vi "Configure Load to Sequence - Single.vi"(8 "error in":errorcluster, 10 "measurement configuration":T6 {"Measurement timeout" format="%.3p"; "Load device voltage/current rating" format="%#_6pA"; "Load voltage/current setpoints" format="%#_6p"; "Load output function" items=["DC Voltage"=1006, "DC Current"=1007, "Pulse Voltage"=1049, "Pulse Current"=1050]; "Load sense" items=["Local"=1008, "Remote"=1009]; "Load transient response" items=["Slow"=1041, "Normal"=1038, "Fast"=1039, "Custom"=1042]; "Load current/voltage limit high" format="%#_6p"; "Load current/voltage limit low" format="%#_6p"; "Load current/voltage limit range" format="%#_6p"; "Load voltage/current level range" format="%#_6p"; "Power ON/Source voltage/current setpoints" format="%#_6p"; "Power ON/Source output function" items=["DC Voltage"=1006, "DC Current"=1007, "Pulse Voltage"=1049, "Pulse Current"=1050]; "Power ON/Source sense" items=["Local"=1008, "Remote"=1009]; "Source transient response" items=["Slow"=1041, "Normal"=1038, "Fast"=1039, "Custom"=1042]; "Source current/voltage limit high" format="%#_6p"; "Source current/voltage limit low" format="%#_6p"; "Power ON/Source current/voltage limit range" format="%#_6p"; "Source voltage/current level range" format="%#_6p"}, 11 "Waveform Mode - Control":T1={"Source Ganged Session Out"={"Ganged Config"=enum."Series", "Session List"=[], "Session Mode"=[], "Channel"=[]}, "Load Ganged Session Out"={"Ganged Config"=enum."Series", "Session List"=[], "Session Mode"=[], "Channel"=[]}, "Source Measure Record Length"=0, "Load Measure Record Length"=0, "Source Sequence Name"="", "Load Sequence Name"="", "Source First Sequence Call"=FALSE, "Load First Sequence Call"=FALSE, "Measurement Results"={"Source dt"=[], "Source voltages"=[], "Source currents"=[], "Ganged source voltages"=[], "Ganged source currents"=[0.0], "Load dt"=[], "Load voltages"=[], "Load currents"=[], "Ganged load voltages"=[], "Ganged load currents"=[], "Status"="", "Eload status"=""}, "No. of eload used"=0, "Measurement timeout"=0.0, "Load Source ON/OFF"=enum."SOURCE AND LOAD ON", "Load session out"="", "Source session out"="", "Load channel name"="", "Source channel name"="", "Source ganged/single"=FALSE, "Load ganged/single"=FALSE, "Source Master/Single resource name"="", "Source Slave resource name"=[], "Load Master/Single resource name"="", "Load Slave resource name"=[]}) -> (0 "error out":errorcluster, 3 "Waveform Mode - Results":T1={"Source Ganged Session Out"={"Ganged Config"=enum."Series", "Session List"=[], "Session Mode"=[], "Channel"=[]}, "Load Ganged Session Out"={"Ganged Config"=enum."Series", "Session List"=[], "Session Mode"=[], "Channel"=[]}, "Source Measure Record Length"=0, "Load Measure Record Length"=0, "Source Sequence Name"="", "Load Sequence Name"="", "Source First Sequence Call"=FALSE, "Load First Sequence Call"=FALSE, "Measurement Results"={"Source dt"=[], "Source voltages"=[], "Source currents"=[], "Ganged source voltages"=[], "Ganged source currents"=[0.0], "Load dt"=[], "Load voltages"=[], "Load currents"=[], "Ganged load voltages"=[], "Ganged load currents"=[], "Status"="", "Eload status"=""}, "No. of eload used"=0, "Measurement timeout"=0.0, "Load Source ON/OFF"=enum."SOURCE AND LOAD ON", "Load session out"="", "Source session out"="", "Load channel name"="", "Source channel name"="", "Source ganged/single"=FALSE, "Load ganged/single"=FALSE, "Source Master/Single resource name"="", "Source Slave resource name"=[], "Load Master/Single resource name"="", "Load Slave resource name"=[]})   [LabVIEW 2021, in "Waveform Mode_Channel Ganging.lvlib"]
doc: "Configure load to sequence"
uses:
  Measurement Configuration.ctl
  Controls/Waveform Mode Measurement.ctl
  shared subVIs/ctl/NIDCPower_channel_ganging - ctl - ganged session.ctl
  shared subVIs/ctl/NIDCPower_channel_ganging - ctl - ganged config.ctl
  shared subVIs/ctl/NIDCPower_channel_ganging - ctl - channel mode.ctl
  Measurement Results.ctl
  <instrlib>/niDCPower/nidcpower.llb/niDCPower Source Mode.ctl
  <instrlib>/niDCPower/nidcpower.llb/niDCPower Sequence Attribute Type.ctl
  <instrlib>/niDCPower/nidcpower.llb/niDCPower Create Advanced Sequence Step With Channels.vi
  Waveform Mode_Channel Ganging.lvlib
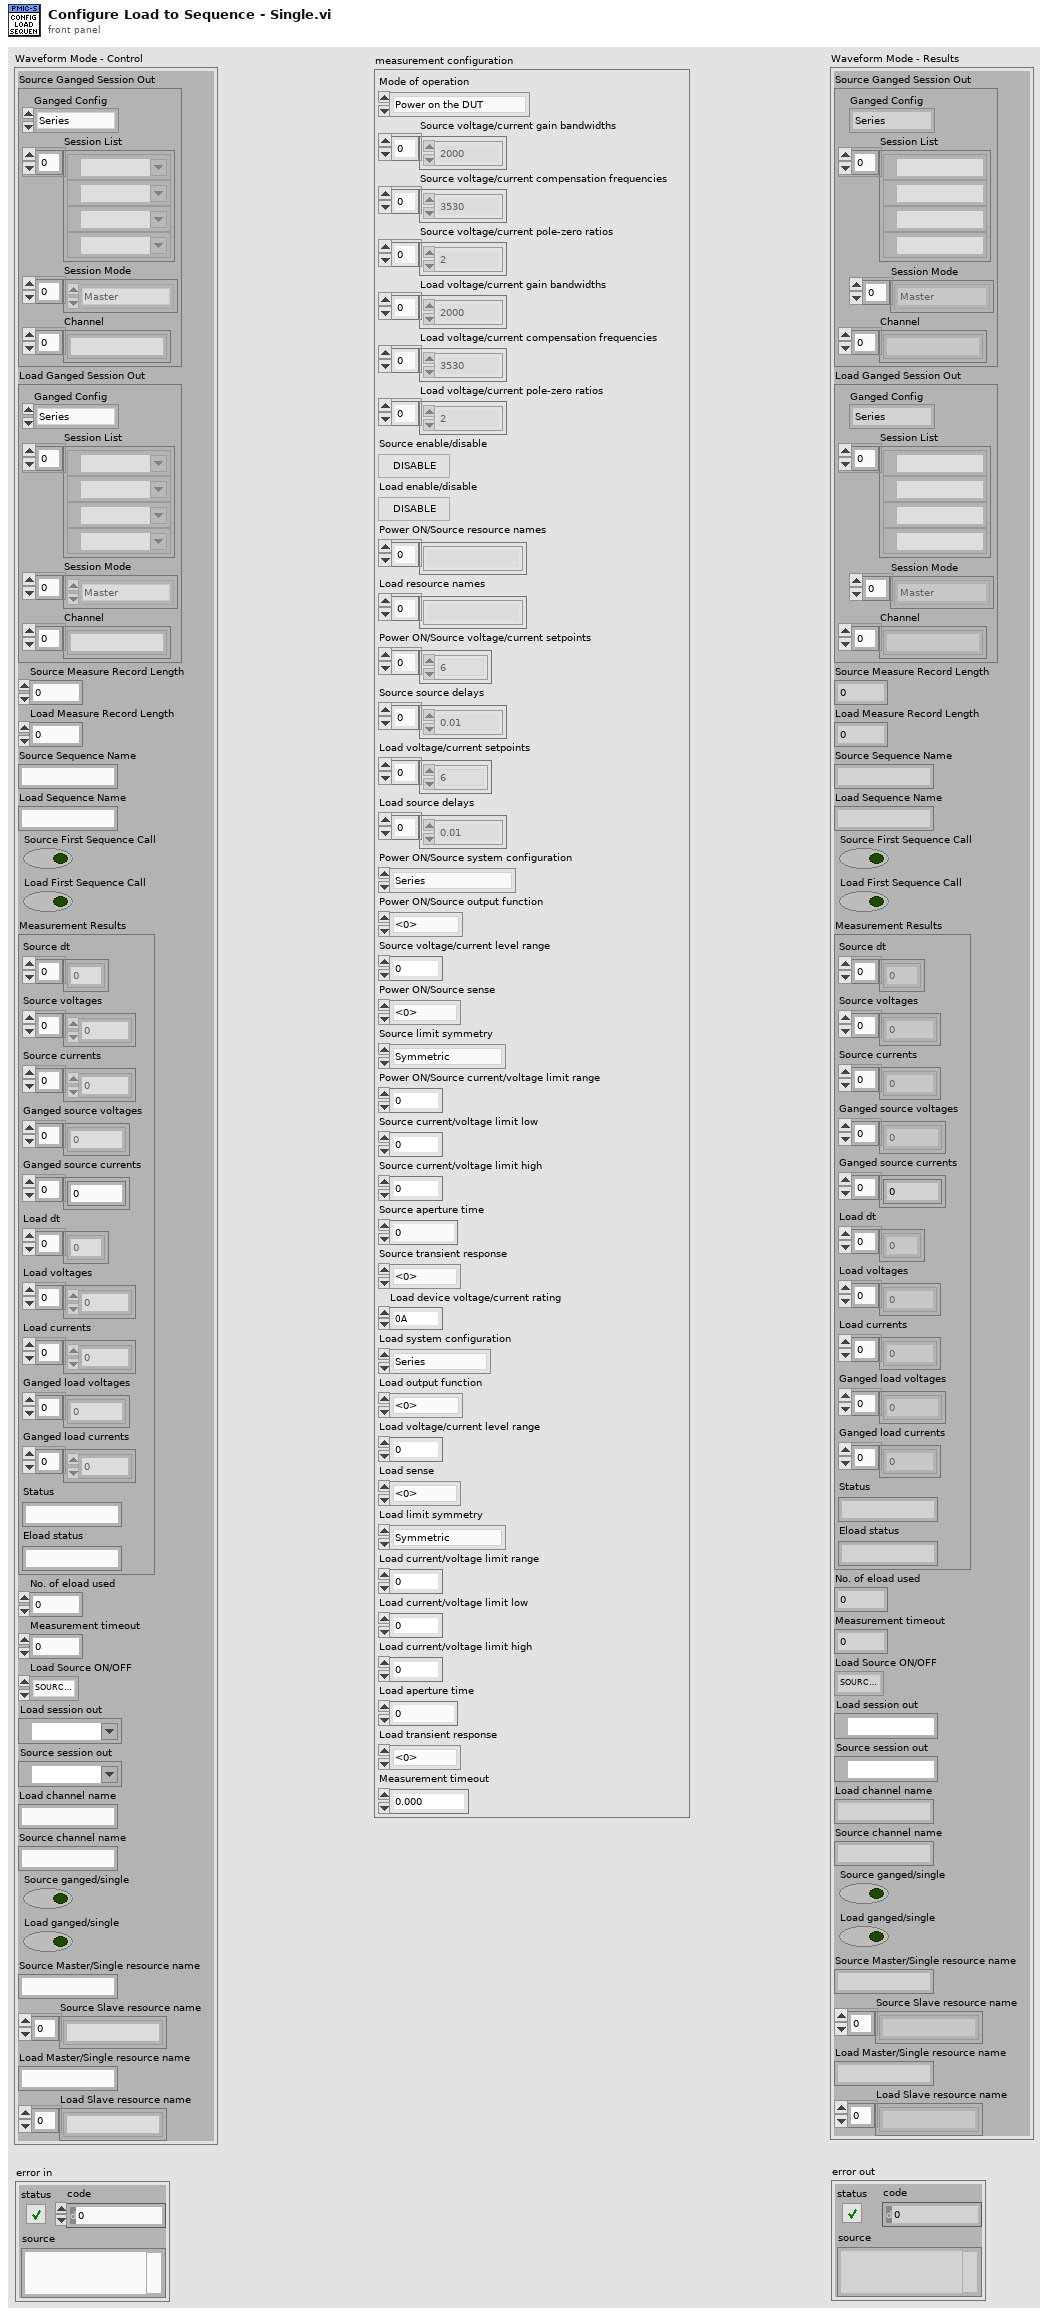
[diagram p1: front panel]
types:
  T1 = typedef "Waveform Mode_Channel Ganging.lvlib/Waveform Mode Measurement.ctl" = cluster{"Source Ganged Session Out":T2, "Load Ganged Session Out":T2, "Source Measure Record Length":i32, "Load Measure Record Length":i32, "Source Sequence Name":string, "Load Sequence Name":string, "Source First Sequence Call":bool, "Load First Sequence Call":bool, "Measurement Results":T5, "No. of eload used":i32, "Measurement timeout":dbl, "Load Source ON/OFF":enum16{"SOURCE AND LOAD OFF", "SOURCE ON", "LOAD ON", "SOURCE AND LOAD ON"}, "Load session out":refnum<k15>, "Source session out":refnum<k15>, "Load channel name":string, "Source channel name":string, "Source ganged/single":bool, "Load ganged/single":bool, "Source Master/Single resource name":string, "Source Slave resource name":string[], "Load Master/Single resource name":string, "Load Slave resource name":string[]}
  T2 = typedef "NIDCPower_channel_ganging - ctl - ganged session.ctl" = cluster{"Ganged Config":T3, "Session List":refnum<k15>[], "Session Mode":T4[], "Channel":string[]}
  T3 = typedef "NIDCPower_channel_ganging - ctl - ganged config.ctl" = enum32{"Series", "Parallel", "Manual"}
  T4 = typedef "NIDCPower_channel_ganging - ctl - channel mode.ctl" = enum32{"Master", "Slave", "Slave - Inverted"}
  T5 = typedef "Waveform Mode_Channel Ganging.lvlib/Measurement Results.ctl" = cluster{"Source dt":dbl[], "Source voltages":dbl[], "Source currents":dbl[], "Ganged source voltages":dbl[], "Ganged source currents":dbl[], "Load dt":dbl[], "Load voltages":dbl[], "Load currents":dbl[], "Ganged load voltages":dbl[], "Ganged load currents":dbl[], "Status":string, "Eload status":string}
  T6 = typedef "Waveform Mode_Channel Ganging.lvlib/Measurement Configuration.ctl" = cluster{"Mode of operation":enum32{"Power on the DUT", "Perform measurement", "Power off the DUT"}, "Source voltage/current gain bandwidths":dbl[], "Source voltage/current compensation frequencies":dbl[], "Source voltage/current pole-zero ratios":dbl[], "Load voltage/current gain bandwidths":dbl[], "Load voltage/current compensation frequencies":dbl[], "Load voltage/current pole-zero ratios":dbl[], "Source enable/disable":bool, "Load enable/disable":bool, "Power ON/Source resource names":string[], "Load resource names":string[], "Power ON/Source voltage/current setpoints":dbl[], "Source source delays":dbl[], "Load voltage/current setpoints":dbl[], "Load source delays":dbl[], "Power ON/Source system configuration":enum32{"Series", "Parallel", "Manual"}, "Power ON/Source output function":i32, "Source voltage/current level range":dbl, "Power ON/Source sense":i32, "Source limit symmetry":enum32{"Symmetric", "Asymmetric"}, "Power ON/Source current/voltage limit range":dbl, "Source current/voltage limit low":dbl, "Source current/voltage limit high":dbl, "Source aperture time":dbl, "Source transient response":i32, "Load device voltage/current rating":dbl, "Load system configuration":enum32{"Series", "Parallel", "Manual"}, "Load output function":i32, "Load voltage/current level range":dbl, "Load sense":i32, "Load limit symmetry":enum32{"Symmetric", "Asymmetric"}, "Load current/voltage limit range":dbl, "Load current/voltage limit low":dbl, "Load current/voltage limit high":dbl, "Load aperture time":dbl, "Load transient response":i32, "Measurement timeout":dbl}
  T7 = typedef "niDCPower Source Mode.ctl" = i32
  T8 = typedef "niDCPower Sequence Attribute Type.ctl" = i32
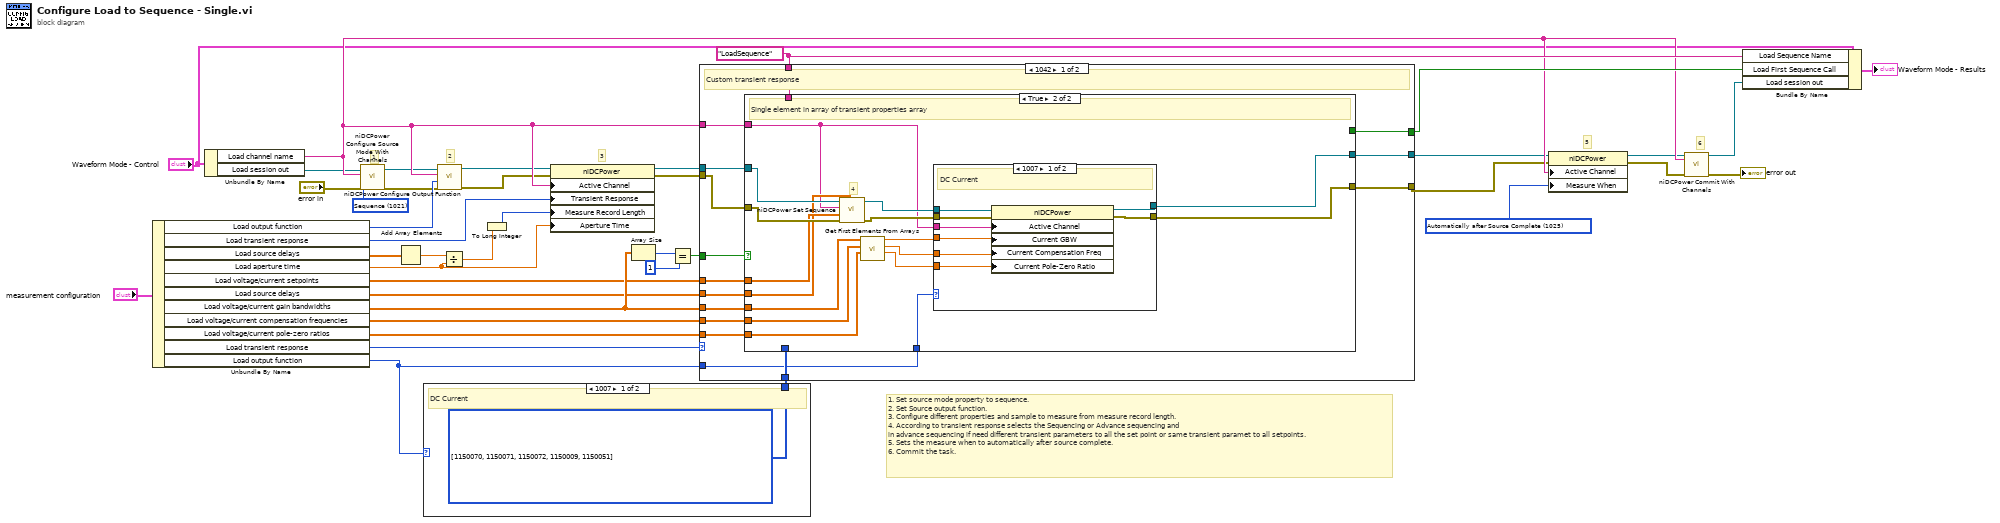
[diagram p0: block diagram]
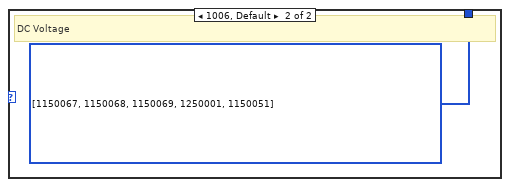
[diagram p2: hidden frame]
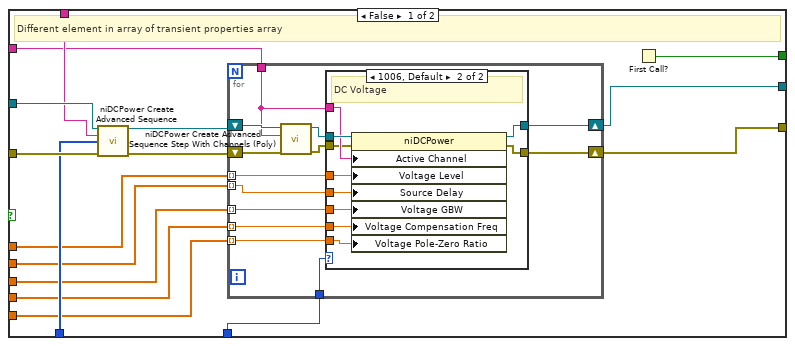
[diagram p3: hidden frame]
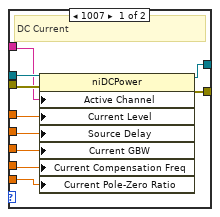
[diagram p4: hidden frame]
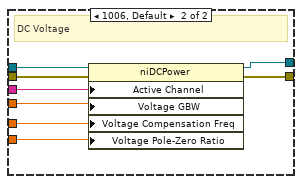
[diagram p5: hidden frame]
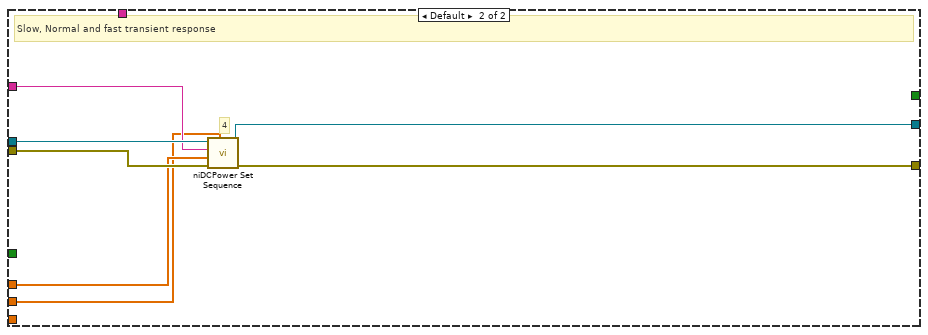
[diagram p6: hidden frame]
diagram:
  w36 = "LoadSequence" ("sequence name")
  w15 = T7 1021 items=["Single Point"=1020, "Sequence"=1021] ("source mode")
  w11 = 1025 items=["Automatically after Source Complete"=1025, "On Demand"=1026, "On Measure Trigger"=1027] ("Measurement:Advanced:Measure When")
  # "1. Set source mode property to sequence.\n2. Set Source output function.\n3. Configure different properties and sample to measure from measure record length.\n4. According to transient response selects the Sequencing or Advance sequencing and\nin advance sequencing if need different transient parameters to all the set point or same transient paramet to all setpoints.\n5. Sets the measure when to automatically after source complete.\n6. Commit the task."
  # "6"
  # "5"
  # "3"
  # "2"
  # "1"
  n1 = Unbundle By Name("measurement configuration") -> ("Load output function"=w20:i32, "Load transient response"=w19:i32, "Load source delays"=w21:dbl[], "Load aperture time"=w29:dbl, "Load voltage/current setpoints"=w17:dbl[], "Load source delays"=w18:dbl[], "Load voltage/current gain bandwidths"=w31:dbl[], "Load voltage/current compensation frequencies"=w27:dbl[], "Load voltage/current pole-zero ratios"=w28:dbl[], "Load transient response"=w25:i32, "Load output function"=w34:i32)
  n2 = Unbundle By Name("Waveform Mode - Control") -> ("Load channel name"=w16:string, "Load session out"=w3:refnum<k15>)
  n3 = call <instrlib>:"niDCPower Configure Source Mode With Channels.vi"("error in (no error)"="error in", "source mode"=w15, "channel name"=w16, "instrument handle"=w3) -> ("error out"=w4:errorcluster, "instrument handle out"=w5:refnum<k15>)  [unwired: 6 in]
  n4 = Add Array Elements(numeric array=w21) -> (sum=w22:dbl)
  n5 = case shown="1007" w34 {
    tunnel: [w41 w42] -> w26
    frame 1007 {
      w41 = T8[] [1150070, 1150071, 1150072, 1150009, 1150051] items=["Source -> Output Function"=1150008, "Source -> Output Enabled"=1250006, "Source -> Output Resistance"=1150061, "Source -> Transient Response"=1150062, "Source -> Custom Transient Response -> Voltage Gain Bandwidth"=1150067, "Source -> Custom Transient Response -> Voltage Compensation Frequency"=1150068, "Source -> Custom Transient Response -> Voltage Pole-Zero Ratio"=1150069, "Source -> Custom Transient Response -> Current Gain Bandwidth"=1150070, "Source -> Custom Transient Response -> Current Compensation Frequency"=1150071, "Source -> Custom Transient Response -> Current Pole-Zero Ratio"=1150072, "Source -> DC Voltage -> Voltage Level"=1250001, "Source -> DC Voltage -> Voltage Level Range"=1150005, "Source -> DC Voltage -> Current Limit"=1250005, "Source -> DC Voltage -> Current Limit High"=1150187, "Source -> DC Voltage -> Current Limit Low"=1150188, "Source -> DC Voltage -> Current Limit Range"=1150004, "Source -> DC Current -> Current Level"=1150009, "Source -> DC Current -> Current Level Range"=1150011, "Source -> DC Current -> Voltage Limit"=1150010, "Source -> DC Current -> Voltage Limit High"=1150185, "Source -> DC Current -> Voltage Limit Low"=1150186, "Source -> DC Current -> Voltage Limit Range"=1150012, "Source -> DC Current -> Current Level Slew Rate -> Rising"=1150343, "Source -> DC Current -> Current Level Slew Rate -> Falling"=1150344, "Source -> Pulse Voltage -> Pulse Voltage Level"=1150080, "Source -> Pulse Voltage -> Pulse Bias Voltage Level"=1150082, "Source -> Pulse Voltage -> Pulse Voltage Level Range"=1150084, "Source -> Pulse Voltage -> Pulse Current Limit"=1150081, "Source -> Pulse Voltage -> Pulse Current Limit High"=1150193, "Source -> Pulse Voltage -> Pulse Current Limit Low"=1150194, "Source -> Pulse Voltage -> Pulse Bias Current Limit"=1150083, "Source -> Pulse Voltage -> Pulse Bias Current Limit High"=1150195, "Source -> Pulse Voltage -> Pulse Bias Current Limit Low"=1150196, "Source -> Pulse Voltage -> Pulse Current Limit Range"=1150085, "Source -> Pulse Current -> Pulse Current Level"=1150086, "Source -> Pulse Current -> Pulse Bias Current Level"=1150088, "Source -> Pulse Current -> Pulse Current Level Range"=1150090, "Source -> Pulse Current -> Pulse Voltage Limit"=1150087, "Source -> Pulse Current -> Pulse Voltage Limit High"=1150189, "Source -> Pulse Current -> Pulse Voltage Limit Low"=1150190, "Source -> Pulse Current -> Pulse Bias Voltage Limit"=1150089, "Source -> Pulse Current -> Pulse Bias Voltage Limit High"=1150191, "Source -> Pulse Current -> Pulse Bias Voltage Limit Low"=1150192, "Source -> Pulse Current -> Pulse Voltage Limit Range"=1150091, "Source -> Advanced -> Source Delay"=1150051, "Source -> Advanced -> Pulse Bias Delay"=1150092, "Source -> Advanced -> Pulse On Time"=1150093, "Source -> Advanced -> Pulse Off Time"=1150094, "Source -> Advanced -> OVP Enabled"=1250002, "Source -> Advanced -> OVP Limit"=1250003, "Source -> Advanced -> Compliance Limit Symmetry"=1150184, "Source -> Advanced -> Sequence Step Delta Time"=1150198, "Source -> Advanced -> Conduction Voltage -> Mode"=1150350, "Source -> Advanced -> Conduction Voltage -> On Threshold"=1150351, "Source -> Advanced -> Conduction Voltage -> Off Threshold"=1150352, "Measurement -> Sense"=1150013, "Measurement -> Aperture Time"=1150058, "Measurement -> Measure Record Length"=1150063, "Measurement -> Advanced -> DC Noise Rejection"=1150066, "Measurement -> Autorange"=1150244, "Measurement -> Advanced -> Autorange Behavior"=1150245, "Measurement -> Advanced -> Autorange Aperture Time Mode"=1150246, "Measurement -> Advanced -> Autorange Minimum Aperture Time"=1150247, "Measurement -> Advanced -> Autorange Minimum Aperture Time Units"=1150248, "Measurement -> Advanced -> Autorange Minimum Current Range"=1150255, "Measurement -> Advanced -> Autorange Minimum Voltage Range"=1150256, "Measurement -> Advanced -> Autorange Threshold Mode"=1150257, "Measurement -> Advanced -> Autorange Maximum Delay After Range Change"=1150322, "LCR -> Instrument Mode"=1150208, "LCR -> Source Delay Mode"=1150315, "LCR -> Measurement Time"=1150218, "LCR -> Custom Measurement Time"=1150258, "LCR -> AC Stimulus -> Function"=1150209, "LCR -> AC Stimulus -> Frequency"=1150210, "LCR -> AC Stimulus -> Voltage Amplitude"=1150211, "LCR -> AC Stimulus -> Current Amplitude"=1150212, "LCR -> AC Stimulus -> Advanced -> Voltage Range"=1150265, "LCR -> AC Stimulus -> Advanced -> Current Range"=1150267, "LCR -> AC Stimulus -> Advanced -> Source Aperture Time"=1150349, "LCR -> DC Bias -> Source"=1150213, "LCR -> DC Bias -> Voltage Level"=1150214, "LCR -> DC Bias -> Current Level"=1150215, "LCR -> DC Bias -> Advanced -> Voltage Range"=1150266, "LCR -> DC Bias -> Advanced -> Current Range"=1150274, "LCR -> DC Bias -> Advanced -> Transient Response"=1150347, "LCR -> Compensation -> Open -> Enabled"=1150220, "LCR -> Compensation -> Open -> Conductance"=1150261, "LCR -> Compensation -> Open -> Susceptance"=1150262, "LCR -> Compensation -> Short -> Enabled"=1150221, "LCR -> Compensation -> Short -> Resistance"=1150263, "LCR -> Compensation -> Short -> Reactance"=1150264, "LCR -> Compensation -> Load -> Enabled"=1150222, "LCR -> Compensation -> Load -> Measured Resistance"=1150268, "LCR -> Compensation -> Load -> Measured Reactance"=1150269, "LCR -> Compensation -> Load -> Actual Resistance"=1150270, "LCR -> Compensation -> Load -> Actual Reactance"=1150271, "LCR -> Impedance Range -> Impedance Range"=1150217, "LCR -> Impedance Range -> Impedance Autorange"=1150216, "LCR -> Impedance Range -> Advanced -> Impedance Range Source"=1150321, "LCR -> Impedance Range -> Advanced -> Load Resistance"=1150318, "LCR -> Impedance Range -> Advanced -> Load Inductance"=1150319, "LCR -> Impedance Range -> Advanced -> Load Capacitance"=1150320] ("advanced sequence properties")
      # "DC Current"
    }
    frame 1006, Default {
      w42 = T8[] [1150067, 1150068, 1150069, 1250001, 1150051] items=["Source -> Output Function"=1150008, "Source -> Output Enabled"=1250006, "Source -> Output Resistance"=1150061, "Source -> Transient Response"=1150062, "Source -> Custom Transient Response -> Voltage Gain Bandwidth"=1150067, "Source -> Custom Transient Response -> Voltage Compensation Frequency"=1150068, "Source -> Custom Transient Response -> Voltage Pole-Zero Ratio"=1150069, "Source -> Custom Transient Response -> Current Gain Bandwidth"=1150070, "Source -> Custom Transient Response -> Current Compensation Frequency"=1150071, "Source -> Custom Transient Response -> Current Pole-Zero Ratio"=1150072, "Source -> DC Voltage -> Voltage Level"=1250001, "Source -> DC Voltage -> Voltage Level Range"=1150005, "Source -> DC Voltage -> Current Limit"=1250005, "Source -> DC Voltage -> Current Limit High"=1150187, "Source -> DC Voltage -> Current Limit Low"=1150188, "Source -> DC Voltage -> Current Limit Range"=1150004, "Source -> DC Current -> Current Level"=1150009, "Source -> DC Current -> Current Level Range"=1150011, "Source -> DC Current -> Voltage Limit"=1150010, "Source -> DC Current -> Voltage Limit High"=1150185, "Source -> DC Current -> Voltage Limit Low"=1150186, "Source -> DC Current -> Voltage Limit Range"=1150012, "Source -> DC Current -> Current Level Slew Rate -> Rising"=1150343, "Source -> DC Current -> Current Level Slew Rate -> Falling"=1150344, "Source -> Pulse Voltage -> Pulse Voltage Level"=1150080, "Source -> Pulse Voltage -> Pulse Bias Voltage Level"=1150082, "Source -> Pulse Voltage -> Pulse Voltage Level Range"=1150084, "Source -> Pulse Voltage -> Pulse Current Limit"=1150081, "Source -> Pulse Voltage -> Pulse Current Limit High"=1150193, "Source -> Pulse Voltage -> Pulse Current Limit Low"=1150194, "Source -> Pulse Voltage -> Pulse Bias Current Limit"=1150083, "Source -> Pulse Voltage -> Pulse Bias Current Limit High"=1150195, "Source -> Pulse Voltage -> Pulse Bias Current Limit Low"=1150196, "Source -> Pulse Voltage -> Pulse Current Limit Range"=1150085, "Source -> Pulse Current -> Pulse Current Level"=1150086, "Source -> Pulse Current -> Pulse Bias Current Level"=1150088, "Source -> Pulse Current -> Pulse Current Level Range"=1150090, "Source -> Pulse Current -> Pulse Voltage Limit"=1150087, "Source -> Pulse Current -> Pulse Voltage Limit High"=1150189, "Source -> Pulse Current -> Pulse Voltage Limit Low"=1150190, "Source -> Pulse Current -> Pulse Bias Voltage Limit"=1150089, "Source -> Pulse Current -> Pulse Bias Voltage Limit High"=1150191, "Source -> Pulse Current -> Pulse Bias Voltage Limit Low"=1150192, "Source -> Pulse Current -> Pulse Voltage Limit Range"=1150091, "Source -> Advanced -> Source Delay"=1150051, "Source -> Advanced -> Pulse Bias Delay"=1150092, "Source -> Advanced -> Pulse On Time"=1150093, "Source -> Advanced -> Pulse Off Time"=1150094, "Source -> Advanced -> OVP Enabled"=1250002, "Source -> Advanced -> OVP Limit"=1250003, "Source -> Advanced -> Compliance Limit Symmetry"=1150184, "Source -> Advanced -> Sequence Step Delta Time"=1150198, "Source -> Advanced -> Conduction Voltage -> Mode"=1150350, "Source -> Advanced -> Conduction Voltage -> On Threshold"=1150351, "Source -> Advanced -> Conduction Voltage -> Off Threshold"=1150352, "Measurement -> Sense"=1150013, "Measurement -> Aperture Time"=1150058, "Measurement -> Measure Record Length"=1150063, "Measurement -> Advanced -> DC Noise Rejection"=1150066, "Measurement -> Autorange"=1150244, "Measurement -> Advanced -> Autorange Behavior"=1150245, "Measurement -> Advanced -> Autorange Aperture Time Mode"=1150246, "Measurement -> Advanced -> Autorange Minimum Aperture Time"=1150247, "Measurement -> Advanced -> Autorange Minimum Aperture Time Units"=1150248, "Measurement -> Advanced -> Autorange Minimum Current Range"=1150255, "Measurement -> Advanced -> Autorange Minimum Voltage Range"=1150256, "Measurement -> Advanced -> Autorange Threshold Mode"=1150257, "Measurement -> Advanced -> Autorange Maximum Delay After Range Change"=1150322, "LCR -> Instrument Mode"=1150208, "LCR -> Source Delay Mode"=1150315, "LCR -> Measurement Time"=1150218, "LCR -> Custom Measurement Time"=1150258, "LCR -> AC Stimulus -> Function"=1150209, "LCR -> AC Stimulus -> Frequency"=1150210, "LCR -> AC Stimulus -> Voltage Amplitude"=1150211, "LCR -> AC Stimulus -> Current Amplitude"=1150212, "LCR -> AC Stimulus -> Advanced -> Voltage Range"=1150265, "LCR -> AC Stimulus -> Advanced -> Current Range"=1150267, "LCR -> AC Stimulus -> Advanced -> Source Aperture Time"=1150349, "LCR -> DC Bias -> Source"=1150213, "LCR -> DC Bias -> Voltage Level"=1150214, "LCR -> DC Bias -> Current Level"=1150215, "LCR -> DC Bias -> Advanced -> Voltage Range"=1150266, "LCR -> DC Bias -> Advanced -> Current Range"=1150274, "LCR -> DC Bias -> Advanced -> Transient Response"=1150347, "LCR -> Compensation -> Open -> Enabled"=1150220, "LCR -> Compensation -> Open -> Conductance"=1150261, "LCR -> Compensation -> Open -> Susceptance"=1150262, "LCR -> Compensation -> Short -> Enabled"=1150221, "LCR -> Compensation -> Short -> Resistance"=1150263, "LCR -> Compensation -> Short -> Reactance"=1150264, "LCR -> Compensation -> Load -> Enabled"=1150222, "LCR -> Compensation -> Load -> Measured Resistance"=1150268, "LCR -> Compensation -> Load -> Measured Reactance"=1150269, "LCR -> Compensation -> Load -> Actual Resistance"=1150270, "LCR -> Compensation -> Load -> Actual Reactance"=1150271, "LCR -> Impedance Range -> Impedance Range"=1150217, "LCR -> Impedance Range -> Impedance Autorange"=1150216, "LCR -> Impedance Range -> Advanced -> Impedance Range Source"=1150321, "LCR -> Impedance Range -> Advanced -> Load Resistance"=1150318, "LCR -> Impedance Range -> Advanced -> Load Inductance"=1150319, "LCR -> Impedance Range -> Advanced -> Load Capacitance"=1150320] ("advanced sequence properties")
      # "DC Voltage"
    }
  }
  n6 = call <instrlib>:"niDCPower Configure Output Function.vi"("error in (no error)"=w4, "output function"=w20, "channel name"=w16, "instrument handle"=w5) -> ("error out"=w7:errorcluster, "instrument handle out"=w6:refnum<k15>)  [unwired: 6 in]
  n7 = Divide(x=w22, y=w29) -> (x/y=w23:dbl)
  n8 = To Long Integer(number=w23) -> (32bit integer=w24:i32)
  n9 = property class="niDCPower"(reference=w6, error in=w7, "Active Channel"=w16, "Transient Response"=w19, "Measure Record Length"=w24, "Aperture Time"=w29) -> (reference out=w8:refnum<k15>, error out=w9:errorcluster)
  n10 = Array Size(array=w31) -> (size(s)=w32:i32)
  n11 = Equal?(x=w32, y=1) -> (x = y?=w33:bool)
  n12 = case shown="1042" w25 {
    tunnel: w8 -> [w57 w145]
    tunnel: w9 -> [w55 w144]
    tunnel: [w54 w143] -> w10
    tunnel: [w53 w142] -> w12
    tunnel: w16 -> [w51 w141]
    tunnel: w17 -> [w50 w140]
    tunnel: w18 -> [w49 w139]
    tunnel: w36 -> [w56 _]
    tunnel: w26 -> [w52 _]
    tunnel: w31 -> [w48 _]
    tunnel: w27 -> [w47 _]
    tunnel: w28 -> [w46 _]
    tunnel: w33 -> [w45 _]
    tunnel: w34 -> [w44 _]
    tunnel: [w43 _] -> w35
    frame 1042 {
      # "Custom transient response"
      n13 = case shown="True" w45 {
        tunnel: w57 -> [w73 w122]
        tunnel: w56 -> [w72 _]
        tunnel: w55 -> [w71 w121]
        tunnel: [w68 w109] -> w54
        tunnel: [w67 w108] -> w53
        tunnel: w52 -> [w66 _]
        tunnel: w51 -> [w65 w116]
        tunnel: w50 -> [w64 w120]
        tunnel: w49 -> [w63 w119]
        tunnel: w48 -> [w62 w115]
        tunnel: w47 -> [w61 w114]
        tunnel: w46 -> [w60 w113]
        tunnel: w44 -> [w59 w107]
        tunnel: [w58 _] -> w43
        frame False {
          # "Different element in array of transient properties array"
          n14 = call <instrlib>:"niDCPower Create Advanced Sequence.vi"("instrument handle"=w73, "sequence name"=w72, "advanced sequence properties"=w66, "error in (no error)"=w71) -> ("instrument handle out"=w70:refnum<k15>, "error out"=w69:errorcluster)  [unwired: 10 in]
          n15 = for {
            shift-right: [w81] -> w67
            shift-left: w69 -> [w86]
            shift-right: [w82] -> w68
            shift-left: w70 -> [w85]
            tunnel: w65 -> [w75]
            tunnel: w64 -> [w80] mode=indexing
            tunnel: w63 -> [w79] mode=indexing
            tunnel: w62 -> [w78] mode=indexing
            tunnel: w61 -> [w77] mode=indexing
            tunnel: w60 -> [w76] mode=indexing
            tunnel: w59 -> [w74]
            n16 = call-poly <instrlib>:"niDCPower Create Advanced Sequence Step With Channels (Poly).vi"("error in (no error)"=w86, "channel name"=w75, "instrument handle"=w85) -> ("error out"=w83:errorcluster, "instrument handle out"=w84:refnum<k15>)  [unwired: 7 in]
            n17 = case shown="1006, Default" w74 {
              tunnel: w84 -> [w96 w106]
              tunnel: w75 -> [w92 w105]
              tunnel: w80 -> [w91 w104]
              tunnel: [w93 w103] -> w82
              tunnel: [w94 w102] -> w81
              tunnel: w83 -> [w95 w101]
              tunnel: w79 -> [w90 w100]
              tunnel: w78 -> [w89 w99]
              tunnel: w77 -> [w88 w98]
              tunnel: w76 -> [w87 w97]
              frame 1007 {
                # "DC Current"
                n18 = property class="niDCPower"(reference=w96, error in=w95, "Active Channel"=w92, "Current Level"=w91, "Source Delay"=w90, "Current GBW"=w89, "Current Compensation Freq"=w88, "Current Pole-Zero Ratio"=w87) -> (reference out=w93:refnum<k15>, error out=w94:errorcluster)
              }
              frame 1006, Default {
                # "DC Voltage"
                n19 = property class="niDCPower"(reference=w106, error in=w101, "Active Channel"=w105, "Voltage Level"=w104, "Source Delay"=w100, "Voltage GBW"=w99, "Voltage Compensation Freq"=w98, "Voltage Pole-Zero Ratio"=w97) -> (reference out=w103:refnum<k15>, error out=w102:errorcluster)
              }
            }
          }
          n20 = First Call?() -> (First Call?: T/F=w58:bool)
        }
        frame True {
          # "4"
          # "Single element in array of transient properties array"
          n21 = call <instrlib>:"niDCPower Set Sequence.vi"("source delays"=w119, "error in (no error)"=w121, "values"=w120, "channel name"=w116, "instrument handle"=w122) -> ("error out"=w117:errorcluster, "instrument handle out"=w118:refnum<k15>)  [unwired: 5 in]
          n22 = call "Get First Elements From Arrays.vi"("Pole-zero ratios"=w113, "Compensation frequencies"=w114, "Gain bandwidths"=w115) -> ("Pole-zero ratio"=w110:dbl, "Compensation frequency"=w111:dbl, "Gain bandwidth"=w112:dbl)  [unwired: 6 in]
          n23 = case shown="1007" w107 {
            tunnel: w117 -> [w130 w138]
            tunnel: [w129 w137] -> w108
            tunnel: w118 -> [w128 w136]
            tunnel: w116 -> [w126 w135]
            tunnel: w112 -> [w127 w134]
            tunnel: w110 -> [w124 w132]
            tunnel: w111 -> [w125 w133]
            tunnel: [w123 w131] -> w109
            frame 1007 {
              # "DC Current"
              n24 = property class="niDCPower"(reference=w128, error in=w130, "Active Channel"=w126, "Current GBW"=w127, "Current Compensation Freq"=w125, "Current Pole-Zero Ratio"=w124) -> (reference out=w123:refnum<k15>, error out=w129:errorcluster)
            }
            frame 1006, Default {
              # "DC Voltage"
              n25 = property class="niDCPower"(reference=w136, error in=w138, "Active Channel"=w135, "Voltage GBW"=w134, "Voltage Compensation Freq"=w133, "Voltage Pole-Zero Ratio"=w132) -> (reference out=w131:refnum<k15>, error out=w137:errorcluster)
            }
          }
        }
      }
    }
    frame Default {
      # "4"
      # "Slow, Normal and fast transient response"
      n26 = call <instrlib>:"niDCPower Set Sequence.vi"("source delays"=w139, "error in (no error)"=w144, "values"=w140, "channel name"=w141, "instrument handle"=w145) -> ("error out"=w142:errorcluster, "instrument handle out"=w143:refnum<k15>)  [unwired: 5 in]
    }
  }
  n27 = property class="niDCPower"(reference=w10, error in=w12, "Active Channel"=w16, "Measure When"=w11) -> (reference out=w13:refnum<k15>, error out=w14:errorcluster)
  n28 = call <instrlib>:"niDCPower Commit With Channels.vi"("error in (no error)"=w14, "channel name"=w16, "instrument handle"=w13) -> ("error out"=→"error out":errorcluster, "instrument handle out"=w37:refnum<k15>)  [unwired: 7 in]
  n29 = Bundle By Name(cluster="Waveform Mode - Control", "Load Sequence Name"=w36, "Load First Sequence Call"=w35, "Load session out"=w37) -> (→"Waveform Mode - Results":T1)
